vi "set ledgen.vi"(0 "WindowHandle in":T1, 2 "Abort Ref":refnum<vi>, 5 "HWND in":u32, 7 "Action":T3(ring), 9 "New val":i32, 11 "error in":errorcluster) -> (4 "WindowHandle out":T1, 6 "HWND out":u32, 8 "Validation Position":T2, 15 "error out":errorcluster)   [LabVIEW 2018]
uses:
  User32.dll
panel:
  # "titlebar: 439, 508\nled 5: 279,550\nled 6: 360, 550\nled 10: 430, 550\nled 13: 500, 550\nled 24: 575, 550\nled 28: 647, 550\nPIN setpoint: 350, 596\nset PIN setpoint: 426, 597\navg points: 354, 627\nset Avg points: 429, 628\nLED freq: 351, 661\nset LED freq: 431, 664\nLED DAC: 351, 694\nset LED DAC: 430, 694\nauto control: 260, 731\nlog to file: 443, 730\nLED Gen ON: 358, 762\nLED Gen OFF: 539, 761"
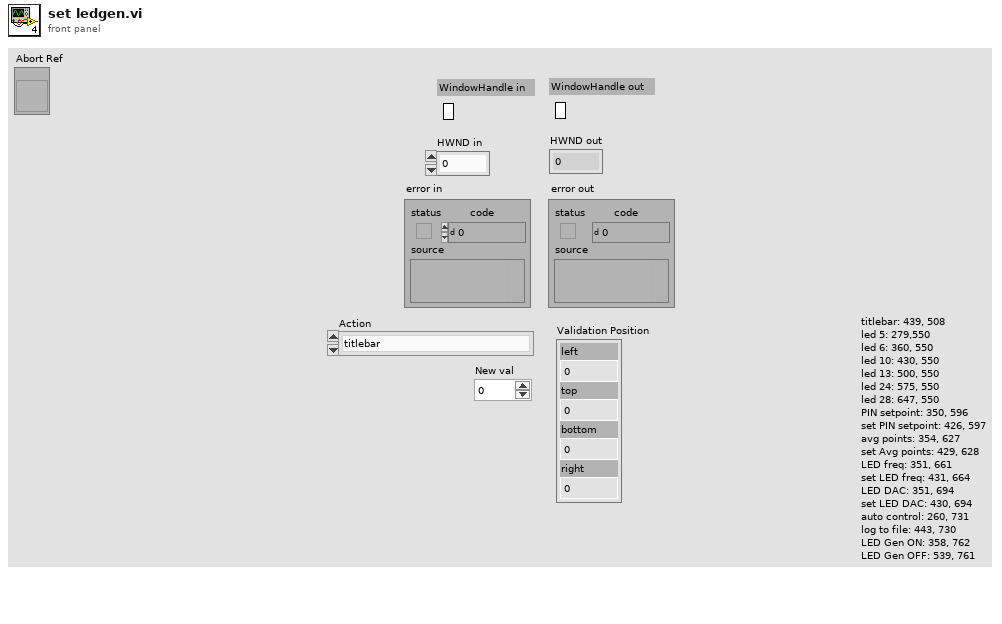
[diagram p1: front panel]
types:
  T1 = typedef "WindowHandle" = refnum<k1>
  T2 = cluster{"left":i32, "top":i32, "bottom":i32, "right":i32}
  T3 = enum16{"titlebar", "led 5", "led 6", "led 10", "led 13", "led 24", "led 28", "set PIN setpoint", "set Avg points", "set LED freq", "set LED DAC", "Toggle auto control", "Toggle Log to File", "LEF Gen ON", "LED Gen Off", "PIN setpoint", "avg points", "LED freq", "LED DAC"}
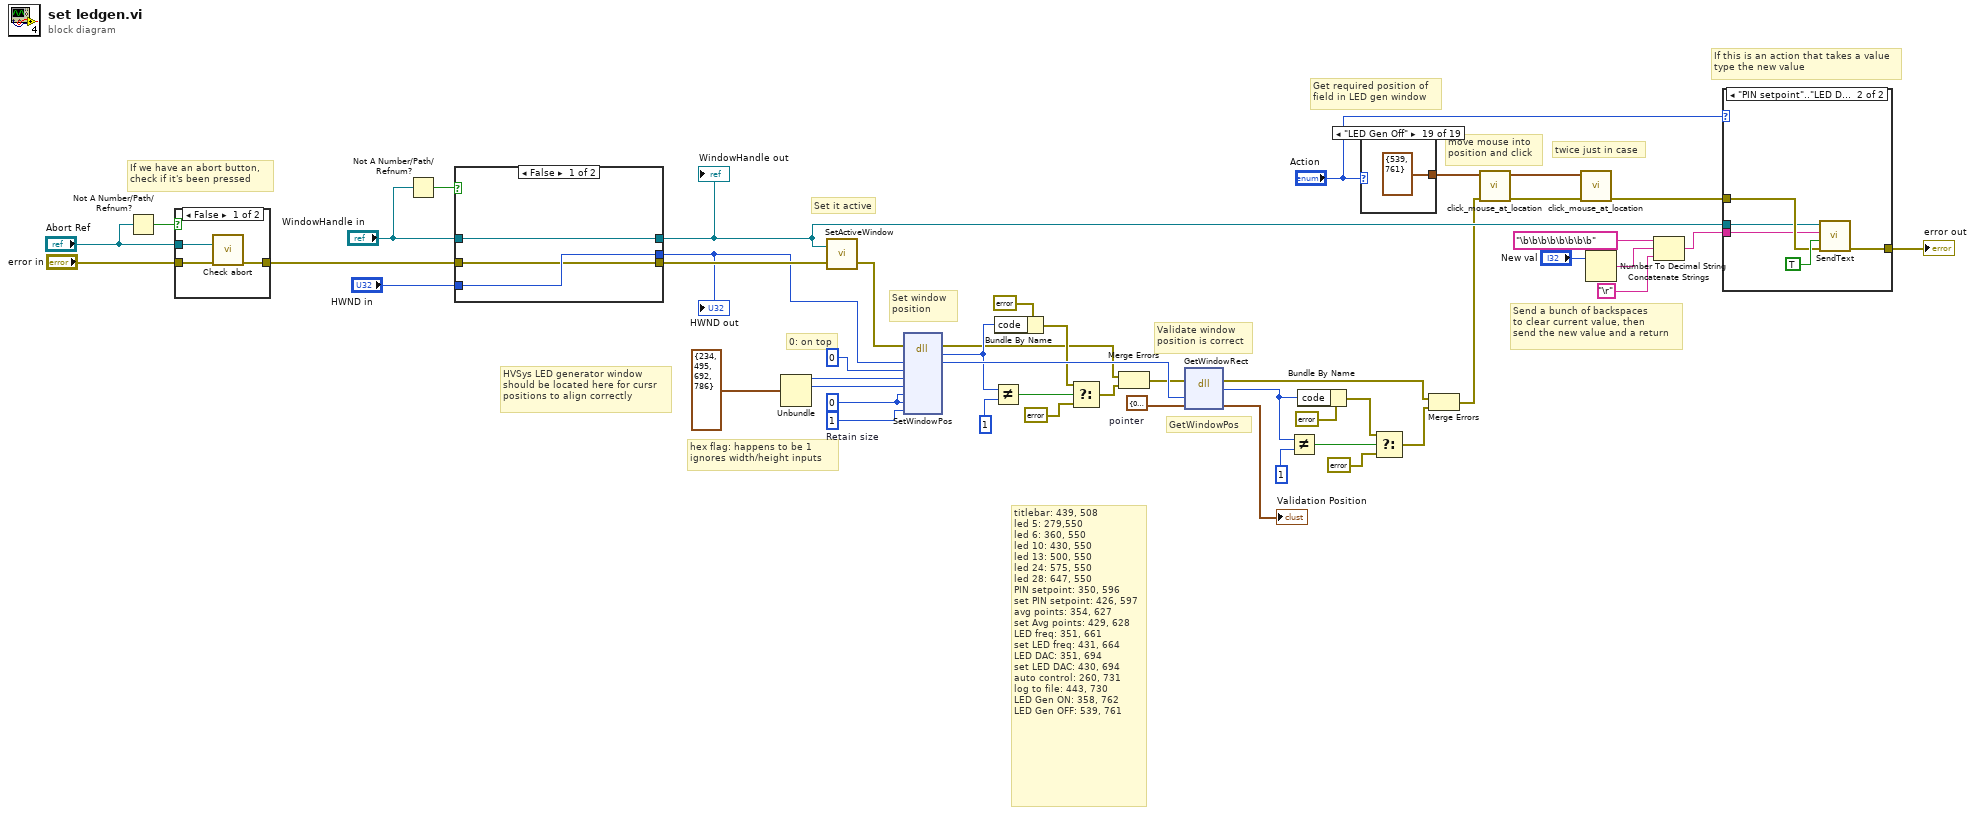
[diagram p0: block diagram]
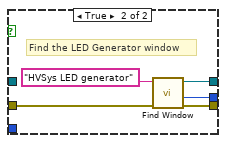
[diagram p3: hidden frame]
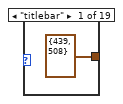
[diagram p5: hidden frame]
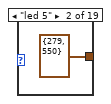
[diagram p6: hidden frame]
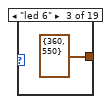
[diagram p7: hidden frame]
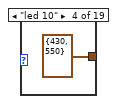
[diagram p8: hidden frame]
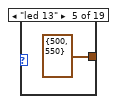
[diagram p9: hidden frame]
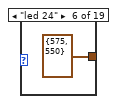
[diagram p10: hidden frame]
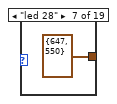
[diagram p11: hidden frame]
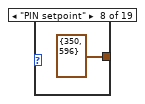
[diagram p12: hidden frame]
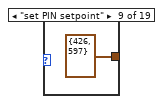
[diagram p13: hidden frame]
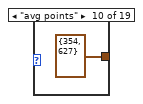
[diagram p14: hidden frame]
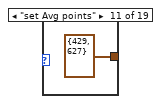
[diagram p15: hidden frame]
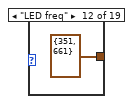
[diagram p16: hidden frame]
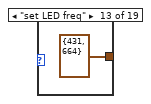
[diagram p17: hidden frame]
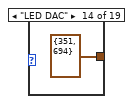
[diagram p18: hidden frame]
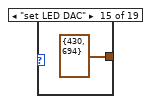
[diagram p19: hidden frame]
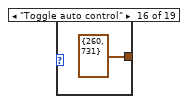
[diagram p20: hidden frame]
diagram:
  w38 = 0 ("height")
  w30 = u32 1  # Retain size
  w41 = T2 {"left"=0, "top"=0, "bottom"=0, "right"=0}  # pointer
  # "If we have an abort button,\ncheck if it's been pressed"
  # "If this is an action that takes a value\ntype the new value"
  # "Send a bunch of backspaces\nto clear current value, then\nsend the new value and a return"
  # "Get required position of\nfield in LED gen window"
  # "Validate window\nposition is correct"
  # "Set window \nposition"
  # "Set it active"
  # "0: on top"
  # "hex flag: happens to be 1\nignores width/height inputs"
  # "HVSys LED generator window\nshould be located here for cursr\npositions to align correctly"
  # "GetWindowPos"
  # "twice just in case"
  # "move mouse into\nposition and click"
  # "titlebar: 439, 508\nled 5: 279,550\nled 6: 360, 550\nled 10: 430, 550\nled 13: 500, 550\nled 24: 575, 550\nled 28: 647, 550\nPIN setpoint: 350, 596\nset PIN setpoint: 426, 597\navg points: 354, 627\nset Avg points: 429, 628\nLED freq: 351, 661\nset LED freq: 431, 664\nLED DAC: 351, 694\nset LED DAC: 430, 694\nauto control: 260, 731\nlog to file: 443, 730\nLED Gen ON: 358, 762\nLED Gen OFF: 539, 761"
  n1 = Not A Number/Path/Refnum?(number/path/refnum="Abort Ref") -> (NaN/Path/Refnum?=w1:bool)
  n2 = case shown="False" w1 {
    tunnel: "error in" -> [w52 w53]
    tunnel: [w51 w53] -> w3
    tunnel: "Abort Ref" -> [w50 _]
    frame False {
      n3 = call "Check abort.vi"("error in (no error)"=w52, "Ctrl Ref in"=w50) -> ("error out"=w51:errorcluster)  [unwired: 7 in, 2 out]
    }
    frame True {
    }
  }
  n4 = Not A Number/Path/Refnum?(number/path/refnum="WindowHandle in") -> (NaN/Path/Refnum?=w7:bool)
  n5 = case shown="False" w7 {
    tunnel: [w54 w60] -> w46
    tunnel: [w56 w59] -> w39
    tunnel: [w55 w58] -> w36
    tunnel: w3 -> [w54 w57]
    tunnel: "WindowHandle in" -> [w56 _]
    tunnel: "HWND in" -> [w55 _]
    frame False {
    }
    frame True {
      # "Find the LED Generator window"
      n6 = call "Find Window.vi"("error in (no error)"=w57, "WindowName"="HVSys LED generator") -> ("error out"=w60:errorcluster, "HWND"=w58:u32, "WindowHandle"=w59:T1)  [unwired: 6 in, 1 out]
    }
  }
  "WindowHandle out" <- w39
  "HWND out" <- w36
  n7 = Unbundle(T2 {"left"=234, "top"=495, "bottom"=692, "right"=786} ("Position")) -> ("left"=w33:i32, "top"=w32:i32)  [unwired: 2 out]
  n8 = call "SetActiveWindow.vi"("error in (no error)"=w46, "WindowHandle"=w39) -> ("error out"=w31:errorcluster)  [unwired: 1 out]
  n9 = dll-call lib="User32.dll" fn="SetWindowPos"(error in=w31, "window handle"=w36, "z pos"=0 ("height"), "left edge"=w33, "top edge"=w32, "width"=w38, "height"=w38, "Flags"=w30) -> (error out=w22:errorcluster, "return"=w28:i32, "window handle"=w35:u32)  [unwired: 8 in, 1 out]
  n10 = Not Equal?(x=w28, y=1 ("Retain size")) -> (x != y?=w26:bool)
  n11 = Bundle By Name(cluster=errorcluster {"status"=TRUE, "code"=0, "source"="Failed to set LEDgen window location!"} ("error out"), "code"=w28) -> (w25:errorcluster)
  n12 = Select(t=w25, s=w26, f=errorcluster {"status"=FALSE, "code"=0, "source"=""}) -> (s? t:f=w23:errorcluster)
  n13 = Merge Errors(w22, w23) -> (w21:errorcluster)
  n14 = dll-call lib="User32.dll" fn="GetWindowRect"(error in=w21, "window handle"=w35, "Position"=w41) -> (error out=w13:errorcluster, "return"=w15:i32, "Position"=→"Validation Position":T2)  [unwired: 3 in, 1 out]
  n15 = Not Equal?(x=w15, y=1 ("Retain size")) -> (x != y?=w18:bool)
  n16 = Bundle By Name(cluster=errorcluster {"status"=TRUE, "code"=0, "source"="Failed to validate LEDgen window location!"} ("error out"), "code"=w15) -> (w19:errorcluster)
  n17 = case shown="\"LED Gen Off\"" "Action" {
    tunnel: [cluster{"x posns":i32, "y posns":i32} {"x posns"=439, "y posns"=508} ("position") cluster{"x posns":i32, "y posns":i32} {"x posns"=279, "y posns"=550} ("position") cluster{"x posns":i32, "y posns":i32} {"x posns"=360, "y posns"=550} ("position") cluster{"x posns":i32, "y posns":i32} {"x posns"=430, "y posns"=550} ("position") cluster{"x posns":i32, "y posns":i32} {"x posns"=500, "y posns"=550} ("position") cluster{"x posns":i32, "y posns":i32} {"x posns"=575, "y posns"=550} ("position") cluster{"x posns":i32, "y posns":i32} {"x posns"=647, "y posns"=550} ("position") cluster{"x posns":i32, "y posns":i32} {"x posns"=350, "y posns"=596} ("position") cluster{"x posns":i32, "y posns":i32} {"x posns"=426, "y posns"=597} ("position") cluster{"x posns":i32, "y posns":i32} {"x posns"=354, "y posns"=627} ("position") cluster{"x posns":i32, "y posns":i32} {"x posns"=429, "y posns"=627} ("position") cluster{"x posns":i32, "y posns":i32} {"x posns"=351, "y posns"=661} ("position") cluster{"x posns":i32, "y posns":i32} {"x posns"=431, "y posns"=664} ("position") cluster{"x posns":i32, "y posns":i32} {"x posns"=351, "y posns"=694} ("position") cluster{"x posns":i32, "y posns":i32} {"x posns"=430, "y posns"=694} ("position") cluster{"x posns":i32, "y posns":i32} {"x posns"=260, "y posns"=731} ("position") cluster{"x posns":i32, "y posns":i32} {"x posns"=443, "y posns"=730} ("position") cluster{"x posns":i32, "y posns":i32} {"x posns"=358, "y posns"=762} ("position") cluster{"x posns":i32, "y posns":i32} {"x posns"=539, "y posns"=761} ("position")] -> w49
    frame "titlebar" {
    }
    frame "led 5" {
    }
    frame "led 6" {
    }
    frame "led 10" {
    }
    frame "led 13" {
    }
    frame "led 24" {
    }
    frame "led 28" {
    }
    frame "PIN setpoint" {
    }
    frame "set PIN setpoint" {
    }
    frame "avg points" {
    }
    frame "set Avg points" {
    }
    frame "LED freq" {
    }
    frame "set LED freq" {
    }
    frame "LED DAC" {
    }
    frame "set LED DAC" {
    }
    frame "Toggle auto control" {
    }
    frame "Toggle Log to File" {
    }
    frame "LEF Gen ON" {
    }
    frame "LED Gen Off" {
    }
  }
  n18 = Select(t=w19, s=w18, f=errorcluster {"status"=FALSE, "code"=0, "source"=""}) -> (s? t:f=w14:errorcluster)
  n19 = Merge Errors(w13, w14) -> (w12:errorcluster)
  n20 = call "click_mouse_at_location.vi"("error in"=w12, "position"=w49) -> ("error out"=w47:errorcluster, "position"=w48:cluster{i32, i32})  [unwired: 8 in]
  n21 = call "click_mouse_at_location.vi"("error in"=w47, "position"=w48) -> ("error out"=w45:errorcluster)  [unwired: 8 in, 1 out]
  n22 = Number To Decimal String(number="New val") -> (decimal integer string=w11:string)  [unwired: 1 in]
  n23 = Concatenate Strings("\b\b\b\b\b\b\b\b" ("Text"), w11, "\r") -> (w43:string)
  n24 = case shown="\"PIN setpoint\"..\"LED DAC\"" "Action" {
    tunnel: w45 -> [w81 w85]
    tunnel: w43 -> [_ w84]
    tunnel: [w81 w83] -> w42
    tunnel: w39 -> [_ w82]
    frame "titlebar".."LED Gen Off" {
    }
    frame "PIN setpoint".."LED DAC" {
      n25 = call "SendText.vi"("error in (no error)"=w85, "Replace LF"=TRUE, "Text"=w84, "WindowHandle"=w82) -> ("error out"=w83:errorcluster)  [unwired: 2 in, 1 out]
    }
  }
  "error out" <- w42
